vi "dust_control_settings_query.vi"(6 "Settings to be loaded":i32=-1, 7 "Query Cluster":T2, 8 "error in (no error)":errorcluster, 9 "Lower Timestamp Range":timestamp=timestamp(3029554800 s since 1904-01-01), 10 "Upper Timestamp Range":timestamp=timestamp(34586550000 s since 1904-01-01), 11 "Settings Type":T1) -> (0 "error out":errorcluster, 3 "Source Control Array":T3[](array[typedef]) {"Needle Voltage" min=0.0 max=10.0 step=0.01 format="%.2g"; "Y Voltage" min=0.0 max=9.0 step=0.01 format="%.2g"; "X Voltage" min=0.0 max=9.0 step=0.01 format="%.2g"; "Einzel Voltage" min=0.0 max=10.0 step=0.01 format="%.2g"; "Desired Amplitude (V)" min=0.0 max=10.0 step=0.01 format="%5.2f"; "Width (ms) : 0.1" min=0.05 max=5.0 step=0.01 format="%6.2f"; "Frequency" min=1.0 max=100.0 step=0.01 format="%.1f"})   [LabVIEW 2013]
doc: "Returns an array of events from the source_settings table based on the tag, dust type, high voltage, and id_source_settings, if specified. Unless a specific id_source_settings is requested, an uppper timestamp range and lower timestamp range are necessary."
uses:
  Controls/dust_soruce_control.ctl
  Controls/Source_settings_select.ctl
  <vilib>/addons/database/_DB Variant To Data/Database Variant To Data.xnode
panel:
  out "SQL Query Syntax":string
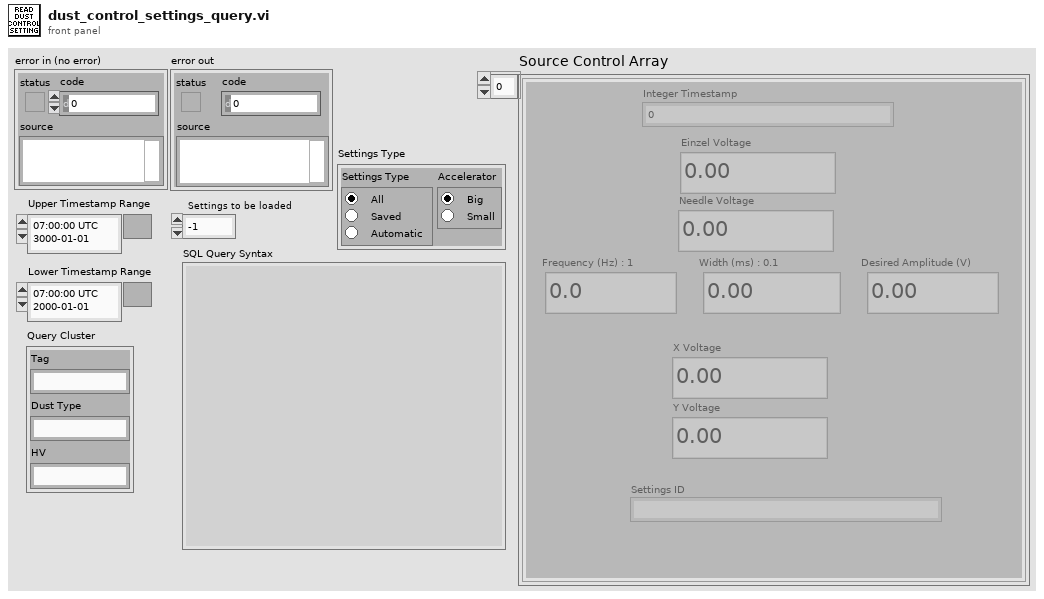
[diagram p1: front panel]
types:
  T1 = typedef "Source_settings_select.ctl" = cluster{"Settings Type":enum32{"All", "Saved", "Automatic"}, "Accelerator":enum32{"Big", "Small"}}
  T2 = cluster{"Tag":string, "Dust Type":string, "HV":string}
  T3 = typedef "dust_soruce_control.ctl" = cluster{"Integer Timestamp":u64, "Einzel Voltage":dbl, "Needle Voltage":dbl, "Frequency":dbl, "Width (ms) : 0.1 ":dbl, "Desired Amplitude (V)":dbl, "X Voltage":dbl, "Y Voltage":dbl, "Settings ID":string, "ID#":i32}
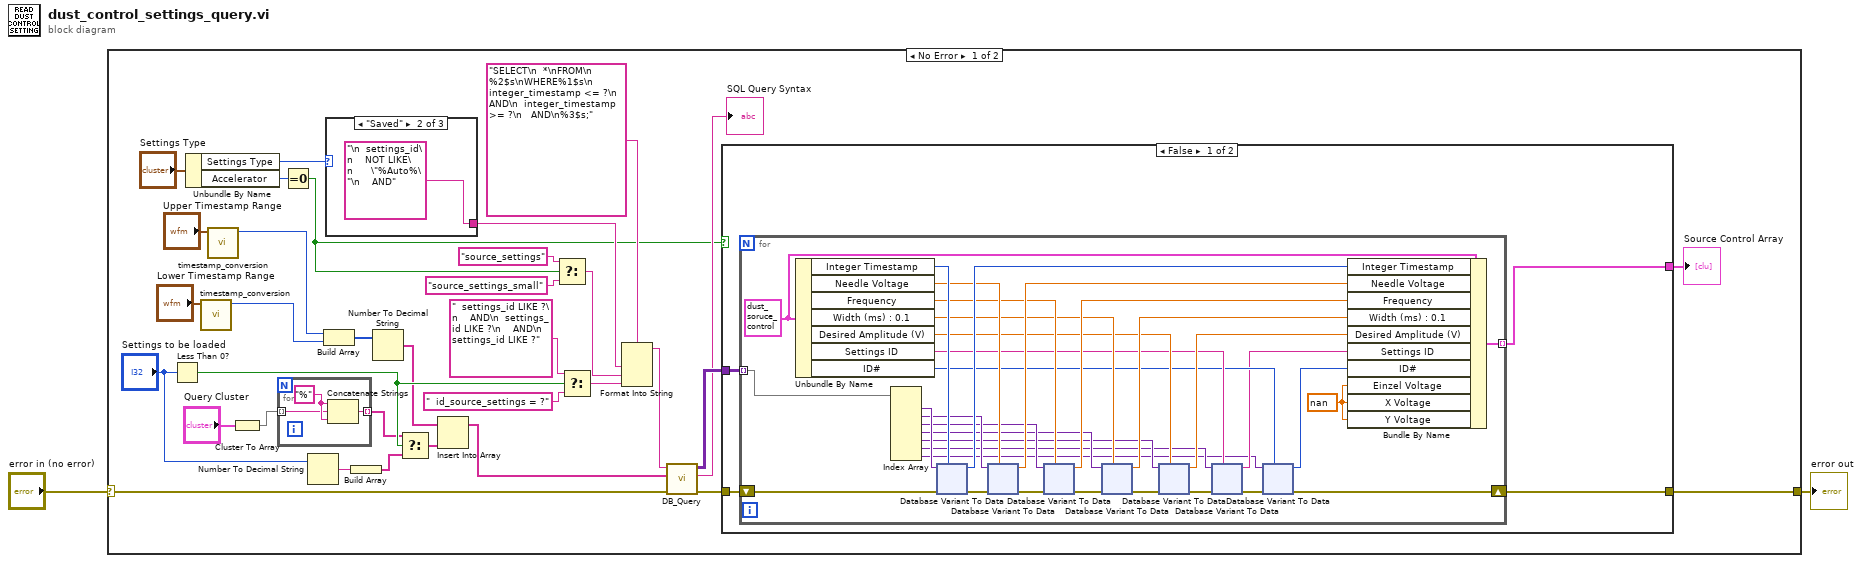
[diagram p0: block diagram]
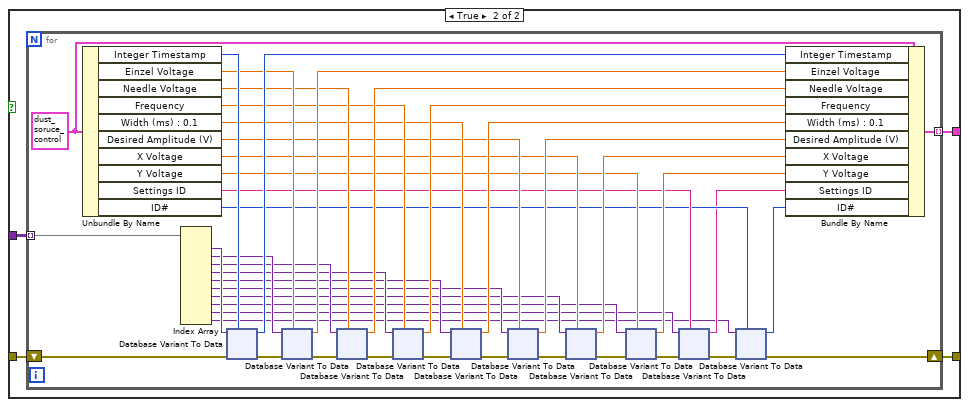
[diagram p2: hidden frame]
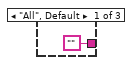
[diagram p3: hidden frame]
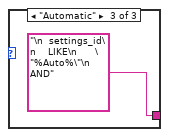
[diagram p4: hidden frame]
diagram:
  n1 = case shown="No Error" "error in (no error)" {
    selector: "error in (no error)" -> [w16 w672]
    tunnel: [w31 w672] -> w1
    frame No Error {
      n2 = Less Than 0?(x="Settings to be loaded") -> (x < 0?=w26:bool)
      n3 = Unbundle By Name("Settings Type") -> ("Settings Type"=w5:enum32{"All", "Saved", "Automatic"}, "Accelerator"=w9:enum32{"Big", "Small"})
      n4 = call "timestamp_conversion.vi"("Time Stamp"="Lower Timestamp Range") -> ("Integer Time"=w27:i64)  [unwired: 8 in, 1 out]
      n5 = call "timestamp_conversion.vi"("Time Stamp"="Upper Timestamp Range") -> ("Integer Time"=w28:i64)  [unwired: 8 in, 1 out]
      n6 = Cluster To Array(cluster="Query Cluster") -> (array=w15:string[])
      n7 = for {
        tunnel: w15 -> [w670] mode=indexing
        tunnel: [w669] -> w14 mode=indexing
        w671 = "%" ("string")
        n8 = Concatenate Strings(w671, w670, w671) -> (w669:string)
      }
      n9 = Equal To 0?(x=w9) -> (x = 0?=w3:bool)
      n10 = Number To Decimal String(number="Settings to be loaded") -> (decimal integer string=w22:string)  [unwired: 1 in]
      n11 = Build Array(w28, w27) -> (w25:i64[])
      n12 = case shown="\"Saved\"" w5 {
        tunnel: ["" "\n  settings_id\n    NOT LIKE\n      \"%Auto%\"\n    AND" "\n  settings_id\n    LIKE\n      \"%Auto%\"\n    AND"] -> w4
        frame "All", Default {
        }
        frame "Saved" {
        }
        frame "Automatic" {
        }
      }
      n13 = Build Array(w22) -> (w21:string[])
      n14 = Number To Decimal String(number=w25) -> (decimal integer string=w20:string[])  [unwired: 1 in]
      n15 = Select(t=w14, s=w26, f=w21) -> (s? t:f=w19:string[])
      n16 = Insert Into Array(array=w20, new element=w19) -> (w17:string[])  [unwired: 1 in]
      n17 = Select(t="source_settings" ("string"), s=w3, f="source_settings_small" ("string")) -> (s? t:f=w6:string)
      n18 = Select(t="  settings_id LIKE ?\n    AND\n  settings_id LIKE ?\n    AND\n  settings_id LIKE ?" ("string"), s=w26, f="  id_source_settings = ?" ("string")) -> (s? t:f=w11:string)
      n19 = Format Into String(format string="SELECT\n  *\nFROM\n  %2$s\nWHERE%1$s\n  integer_timestamp <= ?\n    AND\n  integer_timestamp >= ?\n   AND\n%3$s;" ("string"), w4, w6, w11) -> (resulting string=w12:string)  [unwired: 2 in, 1 out]
      n20 = call "DB_Query.vi"("error in (no error)"=w16, "Parameters"=w17, "Parameterized Query"=w12) -> ("error out"=w32:errorcluster, "Query in Standard Format"=→"SQL Query Syntax":string, "Results"=w33:variant[][])  [unwired: 6 in]
      n21 = case shown="False" w3 {
        tunnel: [w38 w301] -> w34
        tunnel: w33 -> [w37 w300]
        tunnel: w32 -> [w40 w299]
        tunnel: [w39 w298] -> w31
        frame False {
          n22 = for {
            tunnel: w37 -> [w62] mode=indexing
            shift-right: [w53] -> w39
            shift-left: w40 -> [w73]
            tunnel: [w65] -> w38 mode=indexing
            w41 = nan ("Einzel Voltage")
            w63 = T3 {"Integer Timestamp"=0, "Einzel Voltage"=0.0, "Needle Voltage"=0.0, "Frequency"=1.0, "Width (ms) : 0.1 "=0.05, "Desired Amplitude (V)"=0.0, "X Voltage"=0.0, "Y Voltage"=0.0, "Settings ID"="", "ID#"=0} ("Dust Source Controls")
            n23 = Unbundle By Name(w63) -> ("Integer Timestamp"=w61:u64, "Needle Voltage"=w59:dbl, "Frequency"=w58:dbl, "Width (ms) : 0.1"=w57:dbl, "Desired Amplitude (V)"=w56:dbl, "Settings ID"=w55:string, "ID#"=w52:i32)
            n24 = Index Array(array=w62) -> (element #1=w60:variant, element #2=w47:variant, element #3=w46:variant, element #4=w45:variant, element #5=w44:variant, element #6=w43:variant, element #7=w42:variant)  [unwired: 7 in]
            n25 = xnode "Database Variant To Data"("database variant"=w60, "error in (no error)"=w73, "type"=w61) -> ("data"=w64:u64, "error out"=w49:errorcluster)
            n26 = xnode "Database Variant To Data"("database variant"=w47, "error in (no error)"=w49, "type"=w59) -> ("data"=w72:dbl, "error out"=w70:errorcluster)
            n27 = xnode "Database Variant To Data"("database variant"=w46, "error in (no error)"=w70, "type"=w58) -> ("data"=w71:dbl, "error out"=w68:errorcluster)
            n28 = xnode "Database Variant To Data"("database variant"=w45, "error in (no error)"=w68, "type"=w57) -> ("data"=w69:dbl, "error out"=w67:errorcluster)
            n29 = xnode "Database Variant To Data"("database variant"=w44, "error in (no error)"=w67, "type"=w56) -> ("data"=w66:dbl, "error out"=w48:errorcluster)
            n30 = xnode "Database Variant To Data"("database variant"=w43, "error in (no error)"=w48, "type"=w55) -> ("data"=w51:string, "error out"=w54:errorcluster)
            n31 = xnode "Database Variant To Data"("database variant"=w42, "error in (no error)"=w54, "type"=w52) -> ("data"=w50:i32, "error out"=w53:errorcluster)
            n32 = Bundle By Name(cluster=w63, "Integer Timestamp"=w64, "Needle Voltage"=w72, "Frequency"=w71, "Width (ms) : 0.1"=w69, "Desired Amplitude (V)"=w66, "Settings ID"=w51, "ID#"=w50, "Einzel Voltage"=w41, "X Voltage"=w41, "Y Voltage"=w41) -> (w65:T3)
          }
        }
        frame True {
          n33 = for {
            tunnel: w300 -> [w326] mode=indexing
            shift-right: [w306] -> w298
            shift-left: w299 -> [w345]
            tunnel: [w329] -> w301 mode=indexing
            w327 = T3 {"Integer Timestamp"=0, "Einzel Voltage"=0.0, "Needle Voltage"=0.0, "Frequency"=1.0, "Width (ms) : 0.1 "=0.05, "Desired Amplitude (V)"=0.0, "X Voltage"=0.0, "Y Voltage"=0.0, "Settings ID"="", "ID#"=0} ("Dust Source Controls")
            n34 = Unbundle By Name(w327) -> ("Integer Timestamp"=w325:u64, "Einzel Voltage"=w323:dbl, "Needle Voltage"=w321:dbl, "Frequency"=w319:dbl, "Width (ms) : 0.1"=w317:dbl, "Desired Amplitude (V)"=w314:dbl, "X Voltage"=w312:dbl, "Y Voltage"=w311:dbl, "Settings ID"=w309:string, "ID#"=w305:i32)
            n35 = Index Array(array=w326) -> (element #1=w324:variant, element #2=w322:variant, element #3=w320:variant, element #4=w318:variant, element #5=w316:variant, element #6=w315:variant, element #7=w313:variant, element #8=w310:variant, element #9=w308:variant, element #10=w302:variant)  [unwired: 10 in]
            n36 = xnode "Database Variant To Data"("database variant"=w324, "error in"=w345, "type"=w325) -> ("data"=w328:u64, "error out"=w343:errorcluster)
            n37 = xnode "Database Variant To Data"("database variant"=w322, "error in"=w343, "type"=w323) -> ("data"=w344:dbl, "error out"=w341:errorcluster)
            n38 = xnode "Database Variant To Data"("database variant"=w320, "error in"=w341, "type"=w321) -> ("data"=w342:dbl, "error out"=w339:errorcluster)
            n39 = xnode "Database Variant To Data"("database variant"=w318, "error in"=w339, "type"=w319) -> ("data"=w340:dbl, "error out"=w337:errorcluster)
            n40 = xnode "Database Variant To Data"("database variant"=w316, "error in"=w337, "type"=w317) -> ("data"=w338:dbl, "error out"=w336:errorcluster)
            n41 = xnode "Database Variant To Data"("database variant"=w315, "error in"=w336, "type"=w314) -> ("data"=w335:dbl, "error out"=w333:errorcluster)
            n42 = xnode "Database Variant To Data"("database variant"=w313, "error in"=w333, "type"=w312) -> ("data"=w334:dbl, "error out"=w331:errorcluster)
            n43 = xnode "Database Variant To Data"("database variant"=w310, "error in"=w331, "type"=w311) -> ("data"=w332:dbl, "error out"=w330:errorcluster)
            n44 = xnode "Database Variant To Data"("database variant"=w308, "error in"=w330, "type"=w309) -> ("data"=w304:string, "error out"=w307:errorcluster)
            n45 = xnode "Database Variant To Data"("database variant"=w302, "error in (no error)"=w307, "type"=w305) -> ("data"=w303:i32, "error out"=w306:errorcluster)
            n46 = Bundle By Name(cluster=w327, "Integer Timestamp"=w328, "Einzel Voltage"=w344, "Needle Voltage"=w342, "Frequency"=w340, "Width (ms) : 0.1"=w338, "Desired Amplitude (V)"=w335, "X Voltage"=w334, "Y Voltage"=w332, "Settings ID"=w304, "ID#"=w303) -> (w329:T3)
          }
        }
      }
      "Source Control Array" <- w34
    }
    frame Error {
    }
  }
  "error out" <- w1
